vi "Control_Panel_Execute.vi"() -> ()   [LabVIEW 2019]
uses:
  <vilib>/Rock Robotics/WPI/ThirdParty/REV Robotics/SPARK MAX/Typedef/Spark MAX Control Type.ctl
  Globals/Control_Panel_Globals.vi
  Globals/Solenoid Globals.vi
  <vilib>/Rock Robotics/WPI/Solenoid/WPI_SolenoidSetEnum.vi
  <vilib>/Rock Robotics/WPI/Solenoid/WPI_SolenoidValue.ctl
panel:
  in  "time_to_run":u32
  in  "Spinwheel_Throttle":dbl
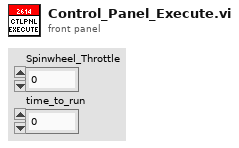
[diagram p1: front panel]
types:
  T1 = typedef "WPI_MotorControlDeviceRef.ctl" = cluster{"DeviceStatus":errorcluster, "Type":T2, "PWM":cluster{"PWM Channel":T3, "DeadBand":T4}, "CAN":cluster{"Device Number":u8, "SetOutput VI Ref":variant, "GetOutput VI Ref":variant, "Enable VI Ref":variant, "Disable VI Ref":variant, "Data":variant}, "Invert":bool, "DIO PWM":cluster{"PWM \"Enable\" Channel":T3, "DIOChannel":T5, "PWM Rate":dbl}}
  T2 = typedef "WPI_MotorControlType.ctl" = enum16{"PWM", "CAN", "DIO PWM"}
  T3 = typedef "FPGA_DIOPWMChannel.ctl" = enum8{"PWM 0", "PWM 1", "PWM 2", "PWM 3", "PWM 4", "PWM 5", "PWM 6", "PWM 7", "PWM 8", "PWM 9", "PWM MXP 0", "PWM MXP 1", "PWM MXP 2", "PWM MXP 3", "PWM MXP 4", "PWM MXP 5", "PWM MXP 6", "PWM MXP 7", "PWM MXP 8", "PWM MXP 9", "Invalid"}
  T4 = typedef "WPI_PWMDeadband.ctl" = cluster{"Name":string, "maxPositivePwm":i32, "minPositivePwm":i32, "centerPwm":i32, "maxNegativePwm":i32, "minNegativePwm":i32, "angularRange":u16}
  T5 = typedef "FPGA_DIOChannel.ctl" = enum8{"DIO 0", "DIO 1", "DIO 2", "DIO 3", "DIO 4", "DIO 5", "DIO 6", "DIO 7", "DIO 8", "DIO 9", "DIO MXP 0", "DIO MXP 1", "DIO MXP 2", "DIO MXP 3", "DIO MXP 4", "DIO MXP 5", "DIO MXP 6", "DIO MXP 7", "DIO MXP 8", "DIO MXP 9", "DIO MXP 10", "DIO MXP 11", "DIO MXP 12", "DIO MXP 13", "DIO MXP 14", "DIO MXP 15", "SPI Port CS1", "SPI Port CS2", "SPI Port CS3", "SPI Port MISO", "SPI Port MOSI", "Invalid"}
  T6 = typedef "WPI_SolenoidDevRef.ctl" = cluster{"DevStatus":errorcluster, "Pneumatics Control Module":u8, "Forward Solenoid Channel":T7, "Reverse Solenoid Channel":T7}
  T7 = typedef "WPI_SolenoidChannel.ctl" = enum8{"Solenoid 0", "Solenoid 1", "Solenoid 2", "Solenoid 3", "Solenoid 4", "Solenoid 5", "Solenoid 6", "Solenoid 7", "Invalid"}
  T8 = typedef "WPI_SolenoidValue.ctl" = enum16{"Off", "On", "Forward", "Reverse"}
  T9 = typedef "Spark MAX Control Type.ctl" = enum16{"Percent VBus", "Voltage", "Velocity", "Position", "Smart Motion", "Current", "Smart Velocity"}
  T10 = typedef "Control_Panel_Cluster.ctl" = cluster{"Control_State":T11, "Start_Movement":bool, "Abort":bool, "Rotation_Control?":bool, "Positional_Control? ":bool, "Throttle":dbl, "Extend?":bool}
  T11 = typedef "Control_Panel_States.ctl" = enum16{"No-Op", "Rotational_Control", "Positional_Control", "Manual_Control"}
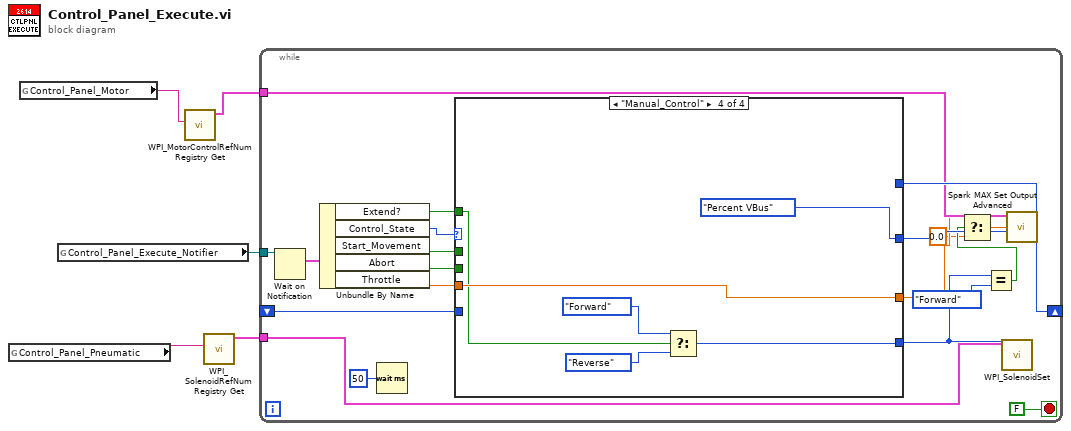
[diagram p0: block diagram]
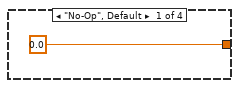
[diagram p2: hidden frame]
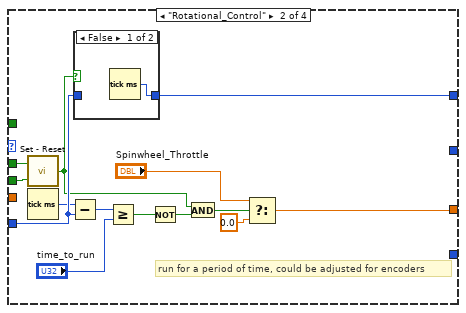
[diagram p3: hidden frame]
diagram:
  n1 = global read "Solenoid Globals.vi" "Control_Panel_Pneumatic"() -> (w4:string)
  n2 = global read "Control_Panel_Globals.vi" "Control_Panel_Motor"() -> (w2:string)
  n3 = global read "Control_Panel_Globals.vi" "Control_Panel_Execute_Notifier"() -> (w5:refnum<notifier>)
  n4 = call <vilib>:"WPI_MotorControlRefNum Registry Get.vi"("refnum name"=w2) -> ("MotorControlDevRef"=w1:T1)  [unwired: 9 in, 1 out]
  n5 = call <vilib>:"WPI_SolenoidRefNum Registry Get.vi"("refnum name"=w4) -> ("SolenoidDevRef"=w3:T6)  [unwired: 9 in, 1 out]
  n6 = while {
    tunnel: w5 -> [w25]
    shift-right: [w20] -> _
    shift-left: _ -> [w19]
    tunnel: w3 -> [w16]
    tunnel: w1 -> [w15]
    stop <- FALSE stop-if-true
    n7 = Wait on Notification(notifier=w25) -> (notification=w24:T10)  [unwired: 3 in, 3 out]
    n8 = Unbundle By Name(w24) -> ("Extend?"=w6:bool, "Control_State"=w13:T11, "Start_Movement"=w22:bool, "Abort"=w21:bool, "Throttle"=w23:dbl)
    n9 = Wait (ms)(milliseconds to wait=u32 50) -> ()  [unwired: 1 out]
    n10 = case shown="\"Manual_Control\"" w13 {
      tunnel: [0.0 ("Spin_Wheel_Speed") w27 _ w48] -> w9
      tunnel: w23 -> [_ _ _ w48]
      tunnel: w22 -> [_ w40 _ _]
      tunnel: w21 -> [_ w39 _ _]
      tunnel: [_ w37 _ _] -> w20
      tunnel: w19 -> [_ w34 _ _]
      tunnel: [_ _ _ Spark_MAX_Control_Type."Percent VBus" ("Control Mode")] -> w14
      tunnel: [_ _ _ w46] -> w7
      tunnel: w6 -> [_ _ _ w45]
      frame "No-Op", Default {
      }
      frame "Rotational_Control" {
        # "run for a period of time, could be adjusted for encoders"
        n11 = call "Set - Reset.vi"("Reset"=w39, "Set"=w40) -> ("Output"=w32:bool)
        n12 = Tick Count (ms)() -> (millisecond timer value=w33:u32)
        n13 = Subtract(x=w33, y=w34) -> (x-y=w36:u32)
        n14 = case shown="False" w32 {
          tunnel: [w41 w42] -> w37
          tunnel: w34 -> [_ w42]
          frame False {
            n15 = Tick Count (ms)() -> (millisecond timer value=w41:u32)
          }
          frame True {
          }
        }
        n16 = Greater Or Equal?(x=w36, y="time_to_run") -> (x >= y?=w31:bool)
        n17 = Not(x=w31) -> (.not. x?=w30:bool)
        n18 = And(x=w32, y=w30) -> (x .and. y?=w29:bool)
        n19 = Select(t="Spinwheel_Throttle", s=w29, f=0.0) -> (s? t:f=w27:dbl)
      }
      frame "Positional_Control" {
        # "SPINNING LOGIC, color offsets"
      }
      frame "Manual_Control" {
        n20 = Select(t=WPI_SolenoidValue."Forward" ("y"), s=w45, f=WPI_SolenoidValue."Reverse" ("y")) -> (s? t:f=w46:T8)
      }
    }
    n21 = Equal?(x=w7, y=WPI_SolenoidValue."Forward") -> (x = y?=w10:bool)
    n22 = Select(t=w9, s=w10, f=0.0) -> (s? t:f=w11:dbl)
    n23 = call-poly <vilib>:"WPI_SolenoidSet.vi"("Value"=w7, "SolenoidDevRef"=w16) -> ()  [unwired: 8 in, 2 out]
    n24 = call <vilib>:"Spark MAX Set Output Advanced.vi"("Control Mode"=w14, "Setpoint"=w11, "MotorControlDevRef"=w15) -> ()  [unwired: 7 in, 2 out]
  }
